vi "Get Inline Buffer.vi"(11 "Transfer in":refnum<class "Transfer.lvclass">) -> (2 "Inline Buffer":refnum<class "Double Pointer.lvclass">, 3 "Transfer out":refnum<class "Transfer.lvclass">)   [LabVIEW 2017, in "Data Sharing Framework Core.lvlib" / "Data Sharing Framework Engine.lvlib" / "Transfer.lvclass"]
uses:
  Transfer.lvclass
  Internal/Memory/Double Pointer/Double Pointer.lvclass
  Transfer.lvclass/Transfer.ctl
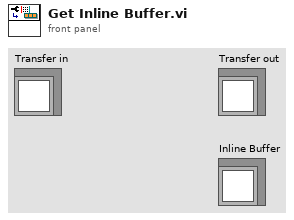
[diagram p1: front panel]
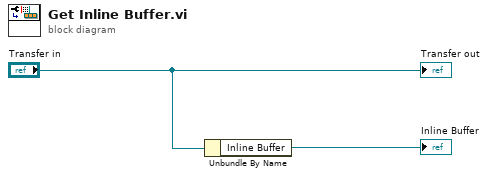
[diagram p0: block diagram]
diagram:
  n1 = Unbundle By Name("Transfer in") -> ("Inline Buffer"=→"Inline Buffer":refnum<class "Double Pointer.lvclass">)
  "Transfer out" <- "Transfer in"
